vi "FT_Write_FT232H_EEPROM.vi"(1 "FT232H EEPROM Contents":T1={"Signature 1"=0, "Signature 2"=4294967295, "Version"=5, "Vendor ID"=1027, "Product ID"=24596, "Manufacturer"="FTDI", "Manufacturer ID"="FT", "Description"="", "Serial Number"="", "Max Power (mA)"=100, "PnP"=0, "Self Powered"=0, "Remote Wake-Up"=0, "Rev4"=0, "Iso In"=0, "Iso Out"=0, "Pull Down Enable"=0, "Serial Number Enable"=0, "USB Version Enable"=0, "USB Version"=512, "Rev5"=0, "Iso In A"=0, "Iso In B"=0, "Iso Out A"=0, "Iso Out B"=0, "Pull Down Enable 5"=0, "Serial Number Enable 5"=0, "USB Version Enable 5"=0, "USB Version 5"=512, "A Is High Current"=0, "B Is High Current"=0, "A Is 245 FIFO"=0, "A Is CPU FIFO"=0, "A Is Fast Serial"=0, "A Is VCP"=0, "B Is 245 FIFO"=0, "B Is CPU FIFO"=0, "B Is Fast Serial"=0, "B Is VCP"=0, "Use Ext Osc"=0, "High Drive IOs"=0, "Endpoint Size"=64, "Pull Down Enable R"=0, "Serial Number Enable R"=0, "Invert TXD"=0, "Invert RXD"=0, "Invert RTS"=0, "Invert CTS"=0, "Invert DTR"=0, "Invert DSR"=0, "Invert DCD"=0, "Invert RI"=0, "CBus0"=0, "CBus1"=0, "CBus2"=0, "CBus3"=0, "CBus4"=5, "R Is VCP"=0, "Pull Down Enable 7"=0, "Serial Number Enable 7"=0, "AL Slow Slew"=0, "AL Schmitt Input"=0, "AL Drive Current"=4, "AH Slow Slew"=0, "AH Schmitt Input"=0, "AH Drive Current"=4, "BL Slow Slew"=0, "BL Schmitt Input"=0, "BL Drive Current"=4, "BH Slow Slew"=0, "BH Schmitt Input"=0, "BH Drive Current"=4, "A Is 245 FIFO 7"=0, "A Is CPU FIFO 7"=0, "A Is Fast Serial 7"=0, "A Is VCP 7"=0, "B Is 245 FIFO 7"=0, "B Is CPU FIFO 7"=0, "B Is Fast Serial 7"=0, "B Is VCP 7"=0, "Power Save"=0, "Pull Down Enable 8"=0, "Serial Number Enable 8"=1, "A Slow Slew"=0, "A Schmitt Input"=0, "A Drive Current"=4, "B Slow Slew"=0, "B Schmitt Input"=0, "B Drive Current"=4, "C Slow Slew"=0, "C Schmitt Input"=0, "C Drive Current"=4, "D Slow Slew"=0, "D Schmitt Input"=0, "D Drive Current"=4, "A RI Is TXDEN"=0, "B RI Is TXDEN"=0, "C RI Is TXDEN"=0, "D RI Is TXDEN"=0, "A Is VCP 8"=1, "B Is VCP 8"=1, "C Is VCP8"=1, "D Is VCP 8"=1, "Pull Down Enable"=0, "Serial Number Enable 9"=0, "AC Slow Slew"=0, "AC Schmitt Input"=0, "AC Drive Current"=4, "AD Slow Slew"=0, "AD Schmitt Input"=0, "AD Drive Current"=4, "CBus0"=0, "CBus1"=0, "CBus2"=0, "CBus3"=0, "CBus4"=0, "CBus5"=0, "CBus6"=0, "CBus7"=0, "CBus8"=0, "CBus9"=0, "Is 245 FIFO"=0, "Is CPU FIFO"=0, "Is Fast Serial"=0, "Is FT1248"=0, "FT1248 Clock Polarity"=0, "FT1248 Bit Order"=0, "FT1248 Flow Control"=0, "Is VCP"=0, "Power Save"=0} {"Power Save" items=["Disabled", "Enabled"]; "Is VCP" items=["D2XX", "VCP"]; "FT1248 Flow Control" items=["Disabled", "Enabled"]; "FT1248 Bit Order" items=["MSB", "LSB"]; "FT1248 Clock Polarity" items=["Idle Low", "Idle High"]; "Is FT1248" items=["Disabled", "Enabled"]; "Is Fast Serial" items=["Disabled", "Enabled"]; "Is CPU FIFO" items=["Disabled", "Enabled"]; "Is 245 FIFO" items=["UART", "FIFO"]; "CBus9" items=["TRISTATE", "RXLED#", "TXLED#", "TX & RXLED#", "PWREN#", "SLEEP#", "DRIVE 0", "DRIVE 1", "IO Mode", "TXDEN#", "30MHz Clock", "15MHz Clock", "7.5MHz Clock"]; "CBus8" items=["TRISTATE", "RXLED#", "TXLED#", "TX & RXLED#", "PWREN#", "SLEEP#", "DRIVE 0", "DRIVE 1", "IO Mode", "TXDEN#", "30MHz Clock", "15MHz Clock", "7.5MHz Clock"]; "CBus7" items=["TRISTATE", "RXLED#", "TXLED#", "TX & RXLED#", "PWREN#", "SLEEP#", "DRIVE 0", "DRIVE 1", "IO Mode", "TXDEN#", "30MHz Clock", "15MHz Clock", "7.5MHz Clock"]; "CBus6" items=["TRISTATE", "RXLED#", "TXLED#", "TX & RXLED#", "PWREN#", "SLEEP#", "DRIVE 0", "DRIVE 1", "IO Mode", "TXDEN#", "30MHz Clock", "15MHz Clock", "7.5MHz Clock"]; "CBus5" items=["TRISTATE", "RXLED#", "TXLED#", "TX & RXLED#", "PWREN#", "SLEEP#", "DRIVE 0", "DRIVE 1", "IO Mode", "TXDEN#", "30MHz Clock", "15MHz Clock", "7.5MHz Clock"]; "CBus4" items=["TRISTATE", "RXLED#", "TXLED#", "TX & RXLED#", "PWREN#", "SLEEP#", "DRIVE 0", "DRIVE 1", "IO Mode", "TXDEN#", "30MHz Clock", "15MHz Clock", "7.5MHz Clock"]; "CBus3" items=["TRISTATE", "RXLED#", "TXLED#", "TX & RXLED#", "PWREN#", "SLEEP#", "DRIVE 0", "DRIVE 1", "IO Mode", "TXDEN#", "30MHz Clock", "15MHz Clock", "7.5MHz Clock"]; "CBus2" items=["TRISTATE", "RXLED#", "TXLED#", "TX & RXLED#", "PWREN#", "SLEEP#", "DRIVE 0", "DRIVE 1", "IO Mode", "TXDEN#", "30MHz Clock", "15MHz Clock", "7.5MHz Clock"]; "CBus1" items=["TRISTATE", "RXLED#", "TXLED#", "TX & RXLED#", "PWREN#", "SLEEP#", "DRIVE 0", "DRIVE 1", "IO Mode", "TXDEN#", "30MHz Clock", "15MHz Clock", "7.5MHz Clock"]; "CBus0" items=["TRISTATE", "RXLED#", "TXLED#", "TX & RXLED#", "PWREN#", "SLEEP#", "DRIVE 0", "DRIVE 1", "IO Mode", "TXDEN#", "30MHz Clock", "15MHz Clock", "7.5MHz Clock"]; "AD Drive Current" items=["4mA"=4, "8mA"=8, "12mA"=12, "16mA"=16]; "AD Schmitt Input" items=["Disabled", "Enabled"]; "AD Slow Slew" items=["Disabled", "Enabled"]; "AC Drive Current" items=["4mA"=4, "8mA"=8, "12mA"=12, "16mA"=16]; "AC Schmitt Input" items=["Disabled", "Enabled"]; "AC Slow Slew" items=["Disabled", "Enabled"]; "Serial Number Enable 9" items=["Disabled", "Enabled"]; "Pull Down Enable" items=["Disabled", "Enabled"]; "D Is VCP 8" items=["D2XX", "VCP"]; "C Is VCP8" items=["D2XX", "VCP"]; "B Is VCP 8" items=["D2XX", "VCP"]; "A Is VCP 8" items=["D2XX", "VCP"]; "D RI Is TXDEN" items=["Disabled", "Enabled"]; "C RI Is TXDEN" items=["Disabled", "Enabled"]; "B RI Is TXDEN" items=["Disabled", "Enabled"]; "A RI Is TXDEN" items=["Disabled", "Enabled"]; "D Drive Current" items=["4mA"=4, "8mA"=8, "12mA"=12, "16mA"=16]; "D Schmitt Input" items=["Disabled", "Enabled"]; "D Slow Slew" items=["Disabled", "Enabled"]; "C Drive Current" items=["4mA"=4, "8mA"=8, "12mA"=12, "16mA"=16]; "C Schmitt Input" items=["Disabled", "Enabled"]; "C Slow Slew" items=["Disabled", "Enabled"]; "B Drive Current" items=["4mA"=4, "8mA"=8, "12mA"=12, "16mA"=16]; "B Schmitt Input" items=["Disabled", "Enabled"]; "B Slow Slew" items=["Disabled", "Enabled"]; "A Drive Current" items=["4mA"=4, "8mA"=8, "12mA"=12, "16mA"=16]; "A Schmitt Input" items=["Disabled", "Enabled"]; "A Slow Slew" items=["Disabled", "Enabled"]; "Serial Number Enable 8" items=["Disabled", "Enabled"]; "Pull Down Enable 8" items=["Disabled", "Enabled"]; "Power Save" items=["Disabled", "Enabled"]; "B Is VCP 7" items=["D2XX", "VCP"]; "B Is Fast Serial 7" items=["Disabled", "Enabled"]; "B Is CPU FIFO 7" items=["Disabled", "Enabled"]; "B Is 245 FIFO 7" items=["UART", "FIFO"]; "A Is VCP 7" items=["D2XX", "VCP"]; "A Is Fast Serial 7" items=["Disabled", "Enabled"]; "A Is CPU FIFO 7" items=["Disabled", "Enabled"]; "A Is 245 FIFO 7" items=["UART", "FIFO"]; "BH Drive Current" items=["4mA"=4, "8mA"=8, "12mA"=12, "16mA"=16]; "BH Schmitt Input" items=["Disabled", "Enabled"]; "BH Slow Slew" items=["Disabled", "Enabled"]; "BL Drive Current" items=["4mA"=4, "8mA"=8, "12mA"=12, "16mA"=16]; "BL Schmitt Input" items=["Disabled", "Enabled"]; "BL Slow Slew" items=["Disabled", "Enabled"]; "AH Drive Current" items=["4mA"=4, "8mA"=8, "12mA"=12, "16mA"=16]; "AH Schmitt Input" items=["Disabled", "Enabled"]; "AH Slow Slew" items=["Disabled", "Enabled"]; "AL Drive Current" items=["4mA"=4, "8mA"=8, "12mA"=12, "16mA"=16]; "AL Schmitt Input" items=["Disabled", "Enabled"]; "AL Slow Slew" items=["Disabled", "Enabled"]; "Serial Number Enable 7" items=["Disabled", "Enabled"]; "Pull Down Enable 7" items=["Disabled", "Enabled"]; "R Is VCP" items=["D2XX", "VCP"]; "CBus4" items=["TXDEN", "PWRON#", "TXLED#", "RXLED#", "TX & RXLED#", "SLEEP#", "48MHz Clock", "24MHz Clock", "12MHz Clock", "6MHz Clock"]; "CBus3" items=["TXDEN", "PWRON#", "TXLED#", "RXLED#", "TX & RXLED#", "SLEEP#", "48MHz Clock", "24MHz Clock", "12MHz Clock", "6MHz Clock", "IO Mode", "Bit-Bang WRn", "Bit-Bang RDn"]; "CBus2" items=["TXDEN", "PWRON#", "TXLED#", "RXLED#", "TX & RXLED#", "SLEEP#", "48MHz Clock", "24MHz Clock", "12MHz Clock", "6MHz Clock", "IO Mode", "Bit-Bang WRn", "Bit-Bang RDn"]; "CBus1" items=["TXDEN", "PWRON#", "TXLED#", "RXLED#", "TX & RXLED#", "SLEEP#", "48MHz Clock", "24MHz Clock", "12MHz Clock", "6MHz Clock", "IO Mode", "Bit-Bang WRn", "Bit-Bang RDn"]; "CBus0" items=["TXDEN", "PWRON#", "TXLED#", "RXLED#", "TX & RXLED#", "SLEEP#", "48MHz Clock", "24MHz Clock", "12MHz Clock", "6MHz Clock", "IO Mode", "Bit-Bang WRn", "Bit-Bang RDn"]; "Invert RI" items=["RI Not Inverted", "RI Inverted"]; "Invert DCD" items=["DCD Not Inverted", "DCD Inverted"]; "Invert DSR" items=["DSR Not Inverted", "DSR Inverted"]; "Invert DTR" items=["DTR Not Inverted", "DTR Inverted"]; "Invert CTS" items=["CTS Not Inverted", "CTS Inverted"]; "Invert RTS" items=["RTS Not Inverted", "RTS Inverted"]; "Invert RXD" items=["RXD Not Inverted", "RXD Inverted"]; "Invert TXD" items=["TXD Not Inverted", "TXD Inverted"]; "Serial Number Enable R" items=["Disabled", "Enabled"]; "Pull Down Enable R" items=["Disabled", "Enabled"]; "Endpoint Size" items=["64"=64, "32"=32, "16"=16, "8"=8, "4"=4]; "High Drive IOs" items=["Disabled", "Enabled"]; "Use Ext Osc" items=["Internal Oscillator", "External Oscillator"]; "B Is VCP" items=["D2XX", "VCP"]; "B Is Fast Serial" items=["Disabled", "Enabled"]; "B Is CPU FIFO" items=["Disabled", "Enabled"]; "B Is 245 FIFO" items=["UART", "FIFO"]; "A Is VCP" items=["D2XX", "VCP"]; "A Is Fast Serial" items=["Disabled", "Enabled"]; "A Is CPU FIFO" items=["Disabled", "Enabled"]; "A Is 245 FIFO" items=["UART", "FIFO"]; "B Is High Current" items=["Disabled", "Enabled"]; "A Is High Current" items=["Disabled", "Enabled"]; "USB Version 5" items=["USB 1.1"=272, "USB 2.0"=512]; "USB Version Enable 5" items=["Disabled", "Enabled"]; "Serial Number Enable 5" items=["Disabled", "Enabled"]; "Pull Down Enable 5" items=["Disabled", "Enabled"]; "Iso Out B" items=["Disabled", "Enabled"]; "Iso Out A" items=["Disabled", "Enabled"]; "Iso In B" items=["Disabled", "Enabled"]; "Iso In A" items=["Disabled", "Enabled"]; "USB Version" items=["USB 1.1"=272, "USB 2.0"=512]; "USB Version Enable" items=["Disabled", "Enabled"]; "Serial Number Enable" items=["Disabled", "Enabled"]; "Pull Down Enable" items=["Disabled", "Enabled"]; "Iso Out" items=["Disabled", "Enabled"]; "Iso In" items=["Disabled", "Enabled"]; "Remote Wake-Up" items=["Disabled", "Enabled"]; "Self Powered" items=["Bus Powered", "Self Powered"]; "PnP" items=["Disabled", "Enabled"]; "Product ID" format="%x"; "Vendor ID" format="%x"; "Signature 2" format="%x"}, 2 "Handle":u32) -> (0 "FT_Status":u32(ring) items=["FT_OK", "FT_INVALID_HANDLE", "FT_DEVICE_NOT_FOUND", "FT_DEVICE_NOT_OPENED", "FT_IO_ERROR", "FT_INSUFFICIENT_RESOURCES", "FT_INVALID_PARAMETER", "FT_INVALID_BAUD_RATE", "FT_DEVICE_NOT_OPENED_FOR_ERASE", "FT_DEVICE_NOT_OPENED_FOR_WRITE", "FT_FAILED_TO_WRITE_DEVICE", "FT_EEPROM_READ_FAILED", "FT_EEPROM_WRITE_FAILED", "FT_EEPROM_ERASE_FAILED", "FT_EEPROM_NOT_PRESENT", "FT_EEPROM_NOT_PROGRAMMED", "FT_INVALID_ARGS", "FT_NOT_SUPPORTED", "FT_OTHER_ERROR"])   [LabVIEW 2010]
uses:
  FTD2XX.dll
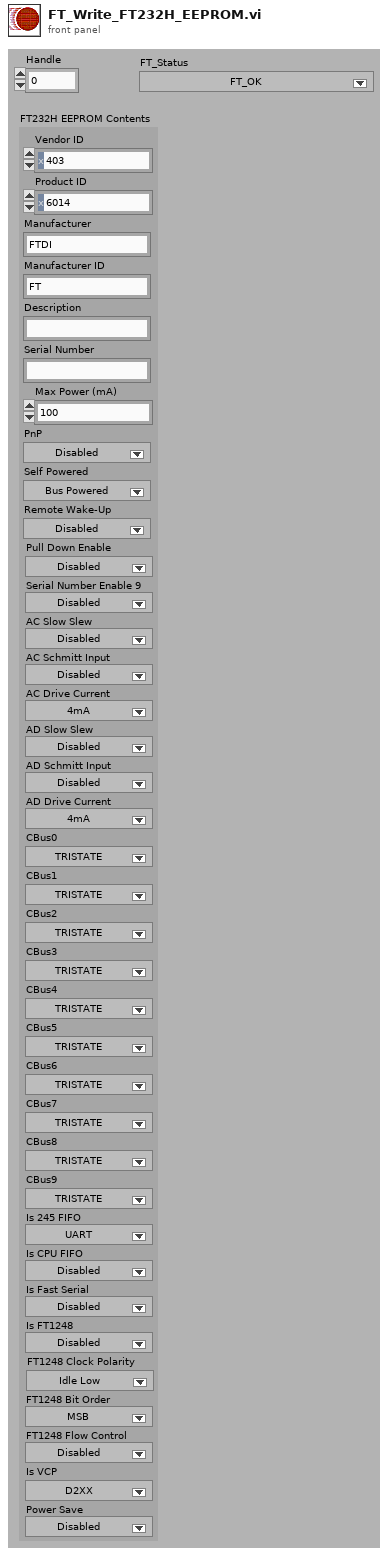
[diagram p1: front panel]
types:
  T1 = cluster{"Signature 1":u32, "Signature 2":u32, "Version":u32, "Vendor ID":u16, "Product ID":u16, "Manufacturer":string, "Manufacturer ID":string, "Description":string, "Serial Number":string, "Max Power (mA)":u16, "PnP":u16, "Self Powered":u16, "Remote Wake-Up":u16, "Rev4":u8, "Iso In":u8, "Iso Out":u8, "Pull Down Enable":u8, "Serial Number Enable":u8, "USB Version Enable":u8, "USB Version":u16, "Rev5":u8, "Iso In A":u8, "Iso In B":u8, "Iso Out A":u8, "Iso Out B":u8, "Pull Down Enable 5":u8, "Serial Number Enable 5":u8, "USB Version Enable 5":u8, "USB Version 5":u16, "A Is High Current":u8, "B Is High Current":u8, "A Is 245 FIFO":u8, "A Is CPU FIFO":u8, "A Is Fast Serial":u8, "A Is VCP":u8, "B Is 245 FIFO":u8, "B Is CPU FIFO":u8, "B Is Fast Serial":u8, "B Is VCP":u8, "Use Ext Osc":u8, "High Drive IOs":u8, "Endpoint Size":u8, "Pull Down Enable R":u8, "Serial Number Enable R":u8, "Invert TXD":u8, "Invert RXD":u8, "Invert RTS":u8, "Invert CTS":u8, "Invert DTR":u8, "Invert DSR":u8, "Invert DCD":u8, "Invert RI":u8, "CBus0":u8, "CBus1":u8, "CBus2":u8, "CBus3":u8, "CBus4":u8, "R Is VCP":u8, "Pull Down Enable 7":u8, "Serial Number Enable 7":u8, "AL Slow Slew":u8, "AL Schmitt Input":u8, "AL Drive Current":u8, "AH Slow Slew":u8, "AH Schmitt Input":u8, "AH Drive Current":u8, "BL Slow Slew":u8, "BL Schmitt Input":u8, "BL Drive Current":u8, "BH Slow Slew":u8, "BH Schmitt Input":u8, "BH Drive Current":u8, "A Is 245 FIFO 7":u8, "A Is CPU FIFO 7":u8, "A Is Fast Serial 7":u8, "A Is VCP 7":u8, "B Is 245 FIFO 7":u8, "B Is CPU FIFO 7":u8, "B Is Fast Serial 7":u8, "B Is VCP 7":u8, "Power Save":u8, "Pull Down Enable 8":u8, "Serial Number Enable 8":u8, "A Slow Slew":u8, "A Schmitt Input":u8, "A Drive Current":u8, "B Slow Slew":u8, "B Schmitt Input":u8, "B Drive Current":u8, "C Slow Slew":u8, "C Schmitt Input":u8, "C Drive Current":u8, "D Slow Slew":u8, "D Schmitt Input":u8, "D Drive Current":u8, "A RI Is TXDEN":u8, "B RI Is TXDEN":u8, "C RI Is TXDEN":u8, "D RI Is TXDEN":u8, "A Is VCP 8":u8, "B Is VCP 8":u8, "C Is VCP8":u8, "D Is VCP 8":u8, "Pull Down Enable":u8, "Serial Number Enable 9":u8, "AC Slow Slew":u8, "AC Schmitt Input":u8, "AC Drive Current":u8, "AD Slow Slew":u8, "AD Schmitt Input":u8, "AD Drive Current":u8, "CBus0":u8, "CBus1":u8, "CBus2":u8, "CBus3":u8, "CBus4":u8, "CBus5":u8, "CBus6":u8, "CBus7":u8, "CBus8":u8, "CBus9":u8, "Is 245 FIFO":u8, "Is CPU FIFO":u8, "Is Fast Serial":u8, "Is FT1248":u8, "FT1248 Clock Polarity":u8, "FT1248 Bit Order":u8, "FT1248 Flow Control":u8, "Is VCP":u8, "Power Save":u8}
  T2 = cluster{"Signature 1":u32, "Signature 2":u32, "Version":u32, "Vendor ID":u16, "Product ID":u16, u32, u32, u32, u32, "Max Power (mA)":u16, "PnP":u16, "Self Powered":u16, "Remote Wake-Up":u16, "Rev4":u8, "Iso In":u8, "Iso Out":u8, "Pull Down Enable":u8, "Serial Number Enable":u8, "USB Version Enable":u8, "USB Version":u16, "Rev5":u8, "Iso In A":u8, "Iso In B":u8, "Iso Out A":u8, "Iso Out B":u8, "Pull Down Enable 5":u8, "Serial Number Enable 5":u8, "USB Version Enable 5":u8, "USB Version 5":u16, "A Is High Current":u8, "B Is High Current":u8, "A Is 245 FIFO":u8, "A Is CPU FIFO":u8, "A Is Fast Serial":u8, "A Is VCP":u8, "B Is 245 FIFO":u8, "B Is CPU FIFO":u8, "B Is Fast Serial":u8, "B Is VCP":u8, "Use Ext Osc":u8, "High Drive IOs":u8, "Endpoint Size":u8, "Pull Down Enable R":u8, "Serial Number Enable R":u8, "Invert TXD":u8, "Invert RXD":u8, "Invert RTS":u8, "Invert CTS":u8, "Invert DTR":u8, "Invert DSR":u8, "Invert DCD":u8, "Invert RI":u8, "CBus0":u8, "CBus1":u8, "CBus2":u8, "CBus3":u8, "CBus4":u8, "R Is VCP":u8, "Pull Down Enable 7":u8, "Serial Number Enable 7":u8, "AL Slow Slew":u8, "AL Schmitt Input":u8, "AL Drive Current":u8, "AH Slow Slew":u8, "AH Schmitt Input":u8, "AH Drive Current":u8, "BL Slow Slew":u8, "BL Schmitt Input":u8, "BL Drive Current":u8, "BH Slow Slew":u8, "BH Schmitt Input":u8, "BH Drive Current":u8, "A Is 245 FIFO 7":u8, "A Is CPU FIFO 7":u8, "A Is Fast Serial 7":u8, "A Is VCP 7":u8, "B Is 245 FIFO 7":u8, "B Is CPU FIFO 7":u8, "B Is Fast Serial 7":u8, "B Is VCP 7":u8, "Power Save":u8, "Pull Down Enable 8":u8, "Serial Number Enable 8":u8, "A Slow Slew":u8, "A Schmitt Input":u8, "A Drive Current":u8, "B Slow Slew":u8, "B Schmitt Input":u8, "B Drive Current":u8, "C Slow Slew":u8, "C Schmitt Input":u8, "C Drive Current":u8, "D Slow Slew":u8, "D Schmitt Input":u8, "D Drive Current":u8, "A RI Is TXDEN":u8, "B RI Is TXDEN":u8, "C RI Is TXDEN":u8, "D RI Is TXDEN":u8, "A Is VCP 8":u8, "B Is VCP 8":u8, "C Is VCP8":u8, "D Is VCP 8":u8, "Pull Down Enable":u8, "Serial Number Enable 9":u8, "AC Slow Slew":u8, "AC Schmitt Input":u8, "AC Drive Current":u8, "AD Slow Slew":u8, "AD Schmitt Input":u8, "AD Drive Current":u8, "CBus0":u8, "CBus1":u8, "CBus2":u8, "CBus3":u8, "CBus4":u8, "CBus5":u8, "CBus6":u8, "CBus7":u8, "CBus8":u8, "CBus9":u8, "Is 245 FIFO":u8, "Is CPU FIFO":u8, "Is Fast Serial":u8, "Is FT1248":u8, "FT1248 Clock Polarity":u8, "FT1248 Bit Order":u8, "FT1248 Flow Control":u8, "Is VCP":u8, "Power Save":u8}
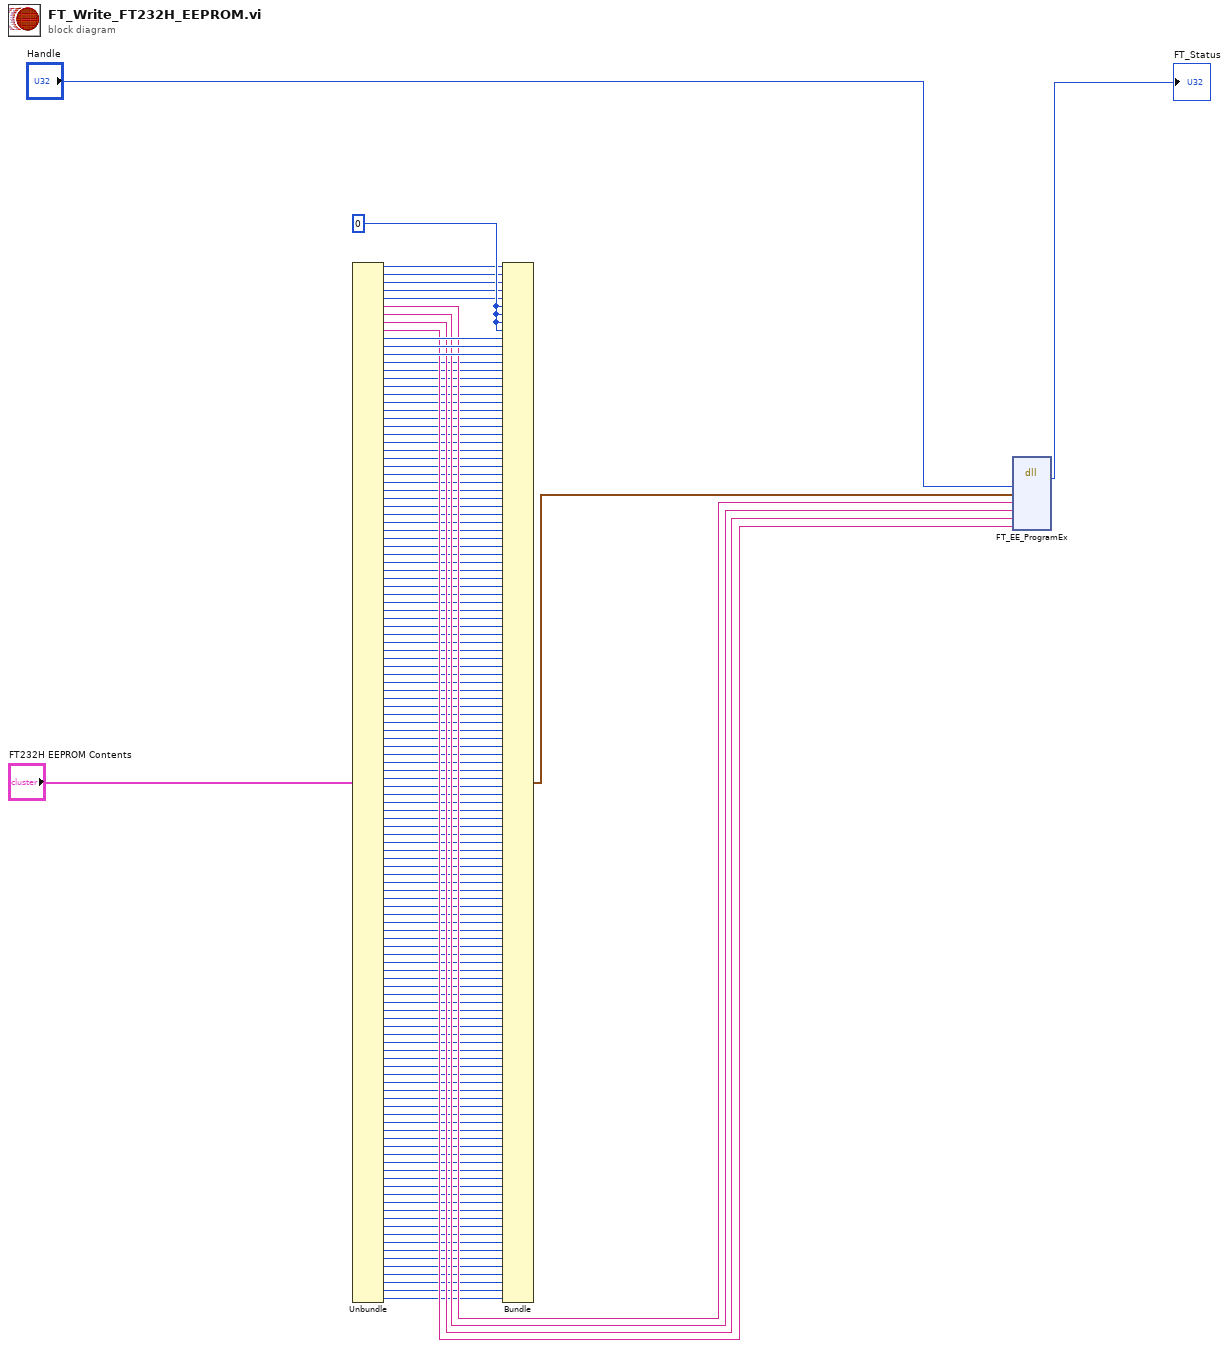
[diagram p0: block diagram]
diagram:
  w133 = u32 0
  n1 = Unbundle("FT232H EEPROM Contents") -> ("Signature 1"=w132:u32, "Signature 2"=w131:u32, "Version"=w130:u32, "Vendor ID"=w129:u16, "Product ID"=w128:u16, "Manufacturer"=w124:string, "Manufacturer ID"=w123:string, "Description"=w122:string, "Serial Number"=w121:string, "Max Power (mA)"=w127:u16, "PnP"=w126:u16, "Self Powered"=w125:u16, "Remote Wake-Up"=w120:u16, "Rev4"=w119:u8, "Iso In"=w118:u8, "Iso Out"=w117:u8, "Pull Down Enable"=w116:u8, "Serial Number Enable"=w115:u8, "USB Version Enable"=w114:u8, "USB Version"=w112:u16, "Rev5"=w113:u8, "Iso In A"=w111:u8, "Iso In B"=w110:u8, "Iso Out A"=w109:u8, "Iso Out B"=w108:u8, "Pull Down Enable 5"=w107:u8, "Serial Number Enable 5"=w106:u8, "USB Version Enable 5"=w105:u8, "USB Version 5"=w104:u16, "A Is High Current"=w103:u8, "B Is High Current"=w102:u8, "A Is 245 FIFO"=w101:u8, "A Is CPU FIFO"=w100:u8, "A Is Fast Serial"=w99:u8, "A Is VCP"=w98:u8, "B Is 245 FIFO"=w97:u8, "B Is CPU FIFO"=w96:u8, "B Is Fast Serial"=w95:u8, "B Is VCP"=w93:u8, "Use Ext Osc"=w94:u8, "High Drive IOs"=w92:u8, "Endpoint Size"=w50:u8, "Pull Down Enable R"=w49:u8, "Serial Number Enable R"=w48:u8, "Invert TXD"=w47:u8, "Invert RXD"=w45:u8, "Invert RTS"=w46:u8, "Invert CTS"=w44:u8, "Invert DTR"=w43:u8, "Invert DSR"=w42:u8, "Invert DCD"=w41:u8, "Invert RI"=w40:u8, "CBus0"=w39:u8, "CBus1"=w38:u8, "CBus2"=w37:u8, "CBus3"=w36:u8, "CBus4"=w35:u8, "R Is VCP"=w34:u8, "Pull Down Enable 7"=w33:u8, "Serial Number Enable 7"=w32:u8, "AL Slow Slew"=w30:u8, "AL Schmitt Input"=w31:u8, "AL Drive Current"=w29:u8, "AH Slow Slew"=w28:u8, "AH Schmitt Input"=w27:u8, "AH Drive Current"=w26:u8, "BL Slow Slew"=w25:u8, "BL Schmitt Input"=w24:u8, "BL Drive Current"=w23:u8, "BH Slow Slew"=w22:u8, "BH Schmitt Input"=w21:u8, "BH Drive Current"=w20:u8, "A Is 245 FIFO 7"=w19:u8, "A Is CPU FIFO 7"=w18:u8, "A Is Fast Serial 7"=w17:u8, "A Is VCP 7"=w16:u8, "B Is 245 FIFO 7"=w15:u8, "B Is CPU FIFO 7"=w14:u8, "B Is Fast Serial 7"=w13:u8, "B Is VCP 7"=w11:u8, "Power Save"=w12:u8, "Pull Down Enable 8"=w10:u8, "Serial Number Enable 8"=w9:u8, "A Slow Slew"=w8:u8, "A Schmitt Input"=w7:u8, "A Drive Current"=w6:u8, "B Slow Slew"=w5:u8, "B Schmitt Input"=w4:u8, "B Drive Current"=w3:u8, "C Slow Slew"=w78:u8, "C Schmitt Input"=w79:u8, "C Drive Current"=w80:u8, "D Slow Slew"=w81:u8, "D Schmitt Input"=w82:u8, "D Drive Current"=w83:u8, "A RI Is TXDEN"=w84:u8, "B RI Is TXDEN"=w85:u8, "C RI Is TXDEN"=w86:u8, "D RI Is TXDEN"=w87:u8, "A Is VCP 8"=w88:u8, "B Is VCP 8"=w89:u8, "C Is VCP8"=w90:u8, "D Is VCP 8"=w91:u8, "Pull Down Enable"=w51:u8, "Serial Number Enable 9"=w52:u8, "AC Slow Slew"=w53:u8, "AC Schmitt Input"=w54:u8, "AC Drive Current"=w55:u8, "AD Slow Slew"=w56:u8, "AD Schmitt Input"=w57:u8, "AD Drive Current"=w58:u8, "CBus0"=w59:u8, "CBus1"=w60:u8, "CBus2"=w61:u8, "CBus3"=w62:u8, "CBus4"=w63:u8, "CBus5"=w64:u8, "CBus6"=w65:u8, "CBus7"=w66:u8, "CBus8"=w67:u8, "CBus9"=w68:u8, "Is 245 FIFO"=w69:u8, "Is CPU FIFO"=w70:u8, "Is Fast Serial"=w71:u8, "Is FT1248"=w73:u8, "FT1248 Clock Polarity"=w72:u8, "FT1248 Bit Order"=w74:u8, "FT1248 Flow Control"=w75:u8, "Is VCP"=w76:u8, "Power Save"=w77:u8)
  n2 = Bundle("Signature 1"=w132, "Signature 2"=w131, "Version"=w130, "Vendor ID"=w129, "Product ID"=w128, w133, w133, w133, w133, "Max Power (mA)"=w127, "PnP"=w126, "Self Powered"=w125, "Remote Wake-Up"=w120, "Rev4"=w119, "Iso In"=w118, "Iso Out"=w117, "Pull Down Enable"=w116, "Serial Number Enable"=w115, "USB Version Enable"=w114, "USB Version"=w112, "Rev5"=w113, "Iso In A"=w111, "Iso In B"=w110, "Iso Out A"=w109, "Iso Out B"=w108, "Pull Down Enable 5"=w107, "Serial Number Enable 5"=w106, "USB Version Enable 5"=w105, "USB Version 5"=w104, "A Is High Current"=w103, "B Is High Current"=w102, "A Is 245 FIFO"=w101, "A Is CPU FIFO"=w100, "A Is Fast Serial"=w99, "A Is VCP"=w98, "B Is 245 FIFO"=w97, "B Is CPU FIFO"=w96, "B Is Fast Serial"=w95, "B Is VCP"=w93, "Use Ext Osc"=w94, "High Drive IOs"=w92, "Endpoint Size"=w50, "Pull Down Enable R"=w49, "Serial Number Enable R"=w48, "Invert TXD"=w47, "Invert RXD"=w45, "Invert RTS"=w46, "Invert CTS"=w44, "Invert DTR"=w43, "Invert DSR"=w42, "Invert DCD"=w41, "Invert RI"=w40, "CBus0"=w39, "CBus1"=w38, "CBus2"=w37, "CBus3"=w36, "CBus4"=w35, "R Is VCP"=w34, "Pull Down Enable 7"=w33, "Serial Number Enable 7"=w32, "AL Slow Slew"=w30, "AL Schmitt Input"=w31, "AL Drive Current"=w29, "AH Slow Slew"=w28, "AH Schmitt Input"=w27, "AH Drive Current"=w26, "BL Slow Slew"=w25, "BL Schmitt Input"=w24, "BL Drive Current"=w23, "BH Slow Slew"=w22, "BH Schmitt Input"=w21, "BH Drive Current"=w20, "A Is 245 FIFO 7"=w19, "A Is CPU FIFO 7"=w18, "A Is Fast Serial 7"=w17, "A Is VCP 7"=w16, "B Is 245 FIFO 7"=w15, "B Is CPU FIFO 7"=w14, "B Is Fast Serial 7"=w13, "B Is VCP 7"=w11, "Power Save"=w12, "Pull Down Enable 8"=w10, "Serial Number Enable 8"=w9, "A Slow Slew"=w8, "A Schmitt Input"=w7, "A Drive Current"=w6, "B Slow Slew"=w5, "B Schmitt Input"=w4, "B Drive Current"=w3, "C Slow Slew"=w78, "C Schmitt Input"=w79, "C Drive Current"=w80, "D Slow Slew"=w81, "D Schmitt Input"=w82, "D Drive Current"=w83, "A RI Is TXDEN"=w84, "B RI Is TXDEN"=w85, "C RI Is TXDEN"=w86, "D RI Is TXDEN"=w87, "A Is VCP 8"=w88, "B Is VCP 8"=w89, "C Is VCP8"=w90, "D Is VCP 8"=w91, "Pull Down Enable"=w51, "Serial Number Enable 9"=w52, "AC Slow Slew"=w53, "AC Schmitt Input"=w54, "AC Drive Current"=w55, "AD Slow Slew"=w56, "AD Schmitt Input"=w57, "AD Drive Current"=w58, "CBus0"=w59, "CBus1"=w60, "CBus2"=w61, "CBus3"=w62, "CBus4"=w63, "CBus5"=w64, "CBus6"=w65, "CBus7"=w66, "CBus8"=w67, "CBus9"=w68, "Is 245 FIFO"=w69, "Is CPU FIFO"=w70, "Is Fast Serial"=w71, "Is FT1248"=w73, "FT1248 Clock Polarity"=w72, "FT1248 Bit Order"=w74, "FT1248 Flow Control"=w75, "Is VCP"=w76, "Power Save"=w77) -> (w135:T2)  [unwired: 1 in]
  n3 = dll-call lib="FTD2XX.dll" fn="FT_EE_ProgramEx" label="FT_EE_WriteEx"("Handle"="Handle", w135, "Manufacturer"=w124, "Manufacturer ID"=w123, "Description"=w122, "Serial Number"=w121) -> ("FT_Status"=→"FT_Status":u32)  [unwired: 9 in, 2 out]
